vi "FireEvent.vi"(9 "event data":cluster{"msg":string, "data":variant}, 10 "EQ_Name":string, 11 "Data Value Reference in":refnum<data-value>) -> (3 "Data Value Reference out":refnum<data-value>)   [LabVIEW 2014]
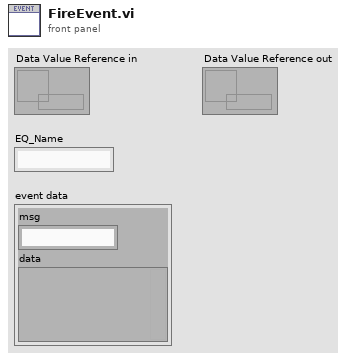
[diagram p1: front panel]
types:
  T1 = cluster{"CmdMsg":cluster{"msg":string, "data":variant}, "EQ_Name":string, "user event out":refnum<user-event>}[]
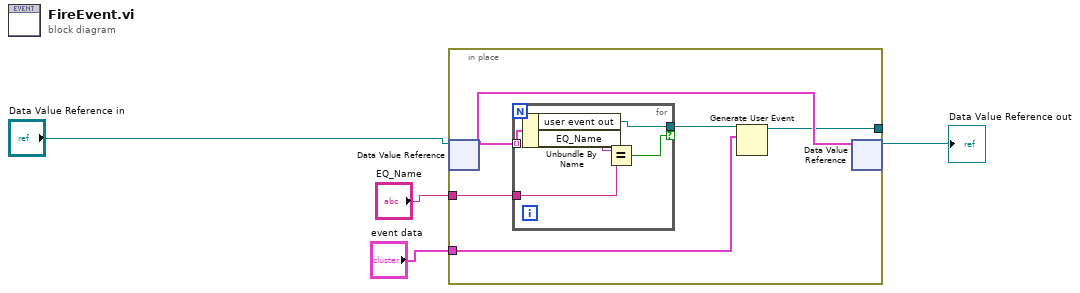
[diagram p0: block diagram]
diagram:
  n1 = in-place {
    in-place-border: [w7] -> _
    in-place-border: "EQ_Name" -> [w6]
    in-place-border: "event data" -> [w5]
    n2 = in-place-dvr #1("Data Value Reference in") -> (w8:T1)  [unwired: 1 out]
    n3 = for {
      tunnel: w8 -> [w14] mode=indexing
      tunnel: [w11] -> w9 if=w12
      tunnel: w6 -> [w10]
      n4 = Unbundle By Name(w14) -> ("user event out"=w11:refnum<user-event>, "EQ_Name"=w13:string)
      n5 = Equal?(x=w13, y=w10) -> (x = y?=w12:bool)
    }
    n6 = Generate User Event(user event=w9, event data cluster=w5) -> (user event out=w7:refnum<user-event>)  [unwired: 2 in, 1 out]
    n7 = in-place-dvr #1(w8) -> (→"Data Value Reference out":refnum<data-value>)  [unwired: 1 out]
  }
